vi "WaitForServerClose.vi"(3 "ROS in":T1={"topic port"=0, "Node"="", "topic"="", "type"="", "node port"=0, "error "={"status"=FALSE, "code"=0, "source"=""}, "Direction"=enum."Node", "APIs"=[], "Update (ms)"=1, "write queue"=1}) -> (0 "Closed":bool, 1 "resulting string":string)   [LabVIEW 2012]
uses:
  SubVIs/_ROSDirection.ctl
  SubVIs/_ROSControl.ctl
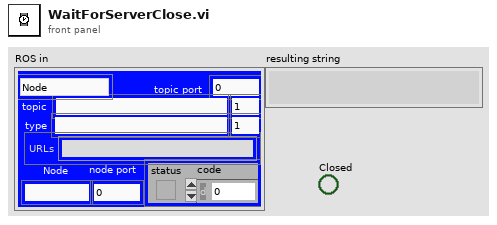
[diagram p1: front panel]
types:
  T1 = typedef "_ROSControl.ctl" = cluster{"topic port":u16, "Node":string, "topic":string, "type":string, "node port":u32, "error ":errorcluster, "Direction":T2, "APIs":string[], "Update (ms)":u16, "write queue":u16}
  T2 = typedef "_ROSDirection.ctl" = enum16{"Node", "Publisher", "Subscriber", "Service Client"}
  T3 = typedef "ServoInfo.ctl" = cluster{"vi name":string, "VI Refnum":refnum<vi>, "queue":refnum<queue>, "ROS":T1, "notifier":refnum<notifier>}
  T4 = enum32{"Bad", "Idle", "Run top level", "Running"}
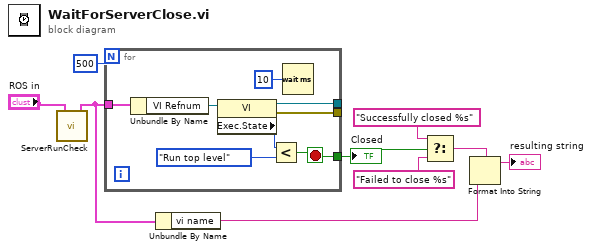
[diagram p0: block diagram]
diagram:
  n1 = call "ServerRunCheck.vi"("ROS in"="ROS in") -> ("ServerFound"=w3:T3)  [unwired: 1 out]
  n2 = for {
    N: 500 -> [_]
    tunnel: w3 -> [w14]
    tunnel: [w13] -> _
    tunnel: [w12] -> w7
    tunnel: [w10] -> _
    stop <- w12 stop-if-true
    n3 = Unbundle By Name(w14) -> ("VI Refnum"=w17:refnum<vi>)
    n4 = property class="VI"(reference=w17) -> (reference out=w10:refnum<vi>, error out=w13:errorcluster, "Exec.State"=w15:T4)  [unwired: 1 in]
    n5 = Less?(x=w15, y=T4."Run top level" ("Execution:State")) -> (x < y?=w12:bool)
    n6 = Wait (ms)(milliseconds to wait=u32 10) -> ()  [unwired: 1 out]
  }
  "Closed" <- w7
  n7 = Unbundle By Name(w3) -> ("vi name"=w2:string)
  n8 = Select(t="Successfully closed %s", s=w7, f="Failed to close %s") -> (s? t:f=w4:string)
  n9 = Format Into String(format string=w4, w2) -> (resulting string=→"resulting string":string)  [unwired: 2 in, 1 out]
